vi "STM Write Message (TCP).vi"(6 "Options":T1={"Ignore Timeout Error"=TRUE, "timeout ms (1000)"=1000}, 8 "error in (no error)":errorcluster, 9 "Data":string, 10 "Name":string, 11 "Connection Info":T2) -> (0 "error out":errorcluster, 3 "Connection Info":T2)   [LabVIEW 2015, in "Diagnostics Addon Engine.lvlib"]
doc: "This VI writes a package of data to a remote computer. It prepends a meta data ID number to each packet. \n\nThe data must be passed in as a String. The calling VI is responsible for flattening the desired data to a string before passing it to this VI."
uses:
  Diagnostics Addon Engine.lvlib
  stm_TCP Connection Info.ctl
  _SubVIs/stm_MetaDataElement.ctl
  stm_TCP Write Options.ctl
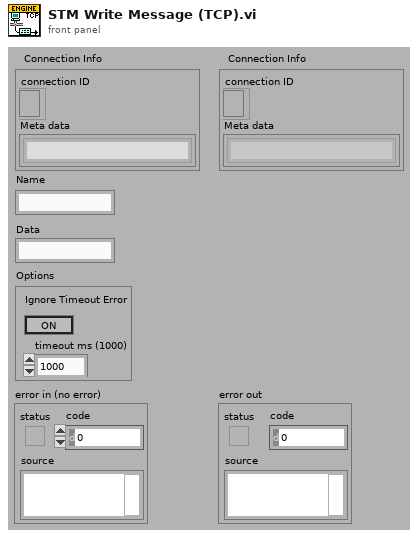
[diagram p1: front panel]
types:
  T1 = typedef "Diagnostics Addon Engine.lvlib/stm_TCP Write Options.ctl" = cluster{"Ignore Timeout Error":bool, "timeout ms (1000)":i32}
  T2 = typedef "Diagnostics Addon Engine.lvlib/stm_TCP Connection Info.ctl" = cluster{"connection ID":refnum<k5>, "Meta data":T3[]}
  T3 = typedef "Diagnostics Addon Engine.lvlib/stm_MetaDataElement.ctl" = string
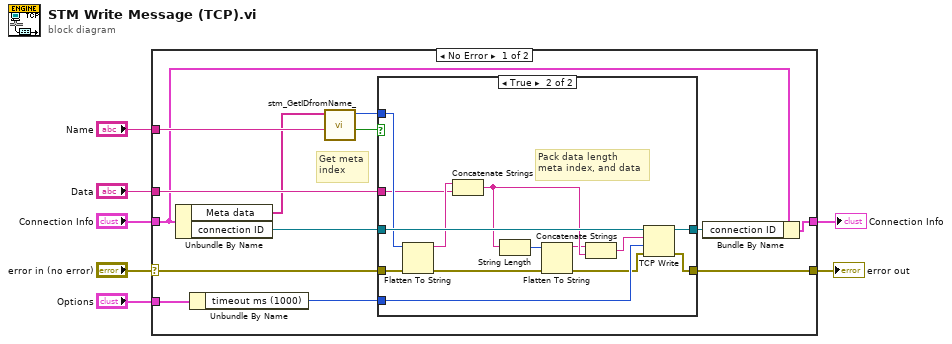
[diagram p0: block diagram]
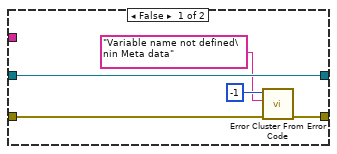
[diagram p2: hidden frame]
diagram:
  n1 = case shown="No Error" "error in (no error)" {
    selector: "error in (no error)" -> [w15 w41]
    tunnel: "Connection Info" -> [w10 w40]
    tunnel: [w20 w41] -> w6
    tunnel: [w9 w40] -> w5
    tunnel: "Name" -> [w19 _]
    tunnel: "Data" -> [w17 _]
    tunnel: "Options" -> [w14 _]
    frame No Error {
      # "Get meta\nindex"
      n2 = Unbundle By Name(w10) -> ("Meta data"=w11:T3[], "connection ID"=w12:refnum<k5>)
      n3 = Unbundle By Name(w14) -> ("timeout ms (1000)"=w13:i32)
      n4 = call "stm_GetIDfromName_.vi"("Name"=w19, "MetaData"=w11) -> ("Found"=w16:bool, "Meta ID"=w18:u16)  [unwired: 8 in]
      n5 = case shown="True" w16 {
        tunnel: w12 -> [w25 w39]
        tunnel: w15 -> [w24 w28]
        tunnel: [w23 w38] -> w20
        tunnel: [w25 w37] -> w8
        tunnel: w18 -> [_ w36]
        tunnel: w17 -> [_ w32]
        tunnel: w13 -> [_ w29]
        frame False {
          n6 = call <vilib>:"Error Cluster From Error Code.vi"("error in (no error)"=w24, "error message (\"\")"="Variable name not defined\nin Meta data" ("source"), "error code (0)"=-1) -> ("error out"=w23:errorcluster)  [unwired: 1 in, 5 out]
        }
        frame True {
          # "Pack data length\nmeta index, and data"
          n7 = Flatten To String(anything=w36, error in (no error)=w28) -> (data string=w35:string, error out=w27:errorcluster)  [unwired: 3 out]
          n8 = Concatenate Strings(w35, w32) -> (w33:string)
          n9 = String Length(string=w33) -> (length=w34:i32)
          n10 = Flatten To String(anything=w34, error in (no error)=w27) -> (data string=w31:string, error out=w26:errorcluster)  [unwired: 3 out]
          n11 = Concatenate Strings(w31, w33) -> (w30:string)
          n12 = TCP Write(connection ID=w39, data in=w30, error in (no error)=w26, 9:w29) -> (connection ID out=w37:refnum<k5>, error out=w38:errorcluster)  [unwired: 1 out]
        }
      }
      n13 = Bundle By Name(cluster=w10, "connection ID"=w8) -> (w9:T2)
    }
    frame Error {
    }
  }
  "error out" <- w6
  "Connection Info" <- w5
